vi "macro_ArmFF_Calculate.vi"   [LabVIEW 2019, in "Trajectory_Library.lvlib"]
uses:
  Trajectory_Library.lvlib
types:
  T1 = typedef "Trajectory_Library.lvlib/ARM_FF.ctl" = cluster{"Ks":dbl, "Kv":dbl, "Ka":dbl, "kCos":dbl}
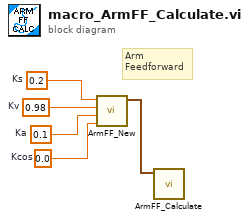
[diagram p0: block diagram]
diagram:
  w2 = 0.2  # Ks
  w3 = 0.98  # Kv
  w4 = 0.1  # Ka
  w5 = 0.0  # Kcos
  # "Arm\nFeedforward"
  n1 = call "ArmFF_New.vi"("Kcos"=w5, "Ka"=w4, "Kv"=w3, "Ks"=w2) -> ("ARM_FF"=w1:T1)  [unwired: 7 in]
  n2 = call "ArmFF_Calculate.vi"("in ARM_FF"=w1) -> ()  [unwired: 10 in, 1 out]
